vi "TCP_CommModule.vi"(8 "error in (no error)":errorcluster) -> (0 "error out":errorcluster)   [LabVIEW 2021]
uses:
  TCPModuleState.ctl
  TCPCommModuleData.ctl
  TCPQueueData.ctl
  ModelQueueCluster.ctl
  ToModelSourceEnum.ctl
  FromTCPCluster.ctl
  ToModelFromTCPMessage.ctl
  FormControllerToMOdelCluster.ctl
  ToModelFromControllerEnum.ctl
  ToSerialCommand.ctl
  ToSerialCTL.ctl
  QueueEnum.ctl
panel:
  out "bytes written":i32
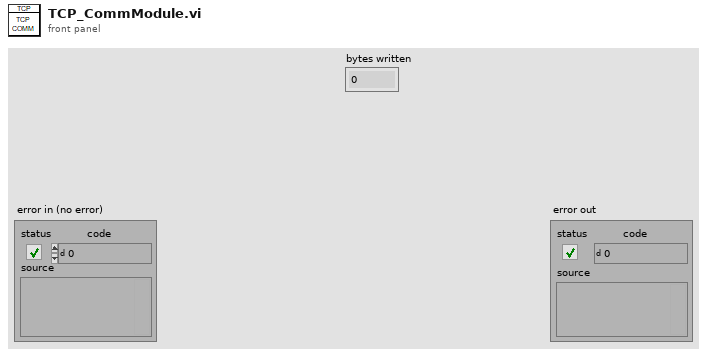
[diagram p1: front panel]
types:
  T1 = typedef "QueueEnum.ctl" = enum16{"Obtain Queue", "Get Queue Ref", "Flush Queue", "Release Queue"}
  T2 = typedef "TCPCommModuleData.ctl" = cluster{"TCP Connection ID":refnum<k5>, "ToTCPModuleQueue":refnum<queue>, "ToModelQueue":refnum<queue>, "Timeout count":u32, "Connected OK?":bool, "ToSerialQueue":refnum<queue>, "VISA resource name":refnum<visa-resource-name>}
  T3 = typedef "TCPModuleState.ctl" = enum16{"Init", "Connect", "Read", "Write", "Disconnect", "ErrorHandler", "Exit"}
  T4 = enum32{"Invalid", "Standard", "Closed", "Hidden", "Minimized", "Maximized"}
  T5 = typedef "TCPQueueData.ctl" = cluster{"Command":T3, "address":string, "remote port":u16, "Data":string}
  T6 = typedef "ModelQueueCluster.ctl" = cluster{"Source":T7, "FromCommunication":T8, "FromControllerCluster":T10}
  T7 = typedef "ToModelSourceEnum.ctl" = enum16{"COM", "TCP", "Controller"}
  T8 = typedef "FromTCPCluster.ctl" = cluster{"Message":T9, "Data":string, "StatusOK?":bool}
  T9 = typedef "ToModelFromTCPMessage.ctl" = enum16{"Exit", "DataWritten", "DataReceived", "Timeout", "UnableToConnect", "Disconnected", "Connected"}
  T10 = typedef "FormControllerToMOdelCluster.ctl" = cluster{"Command":T11, "IP Address":string, "Remote Port":u16, "Data":string, "TCP/COM":bool, "VISA resource name":refnum<visa-resource-name>}
  T11 = typedef "ToModelFromControllerEnum.ctl" = enum16{"StopLogging", "StartLogging", "SlideChange", "SendMessage", "Exit", "Disconnect", "Connect"}
  T12 = enum16{"Standard", "Buffered", "CRLF", "Immediate"}
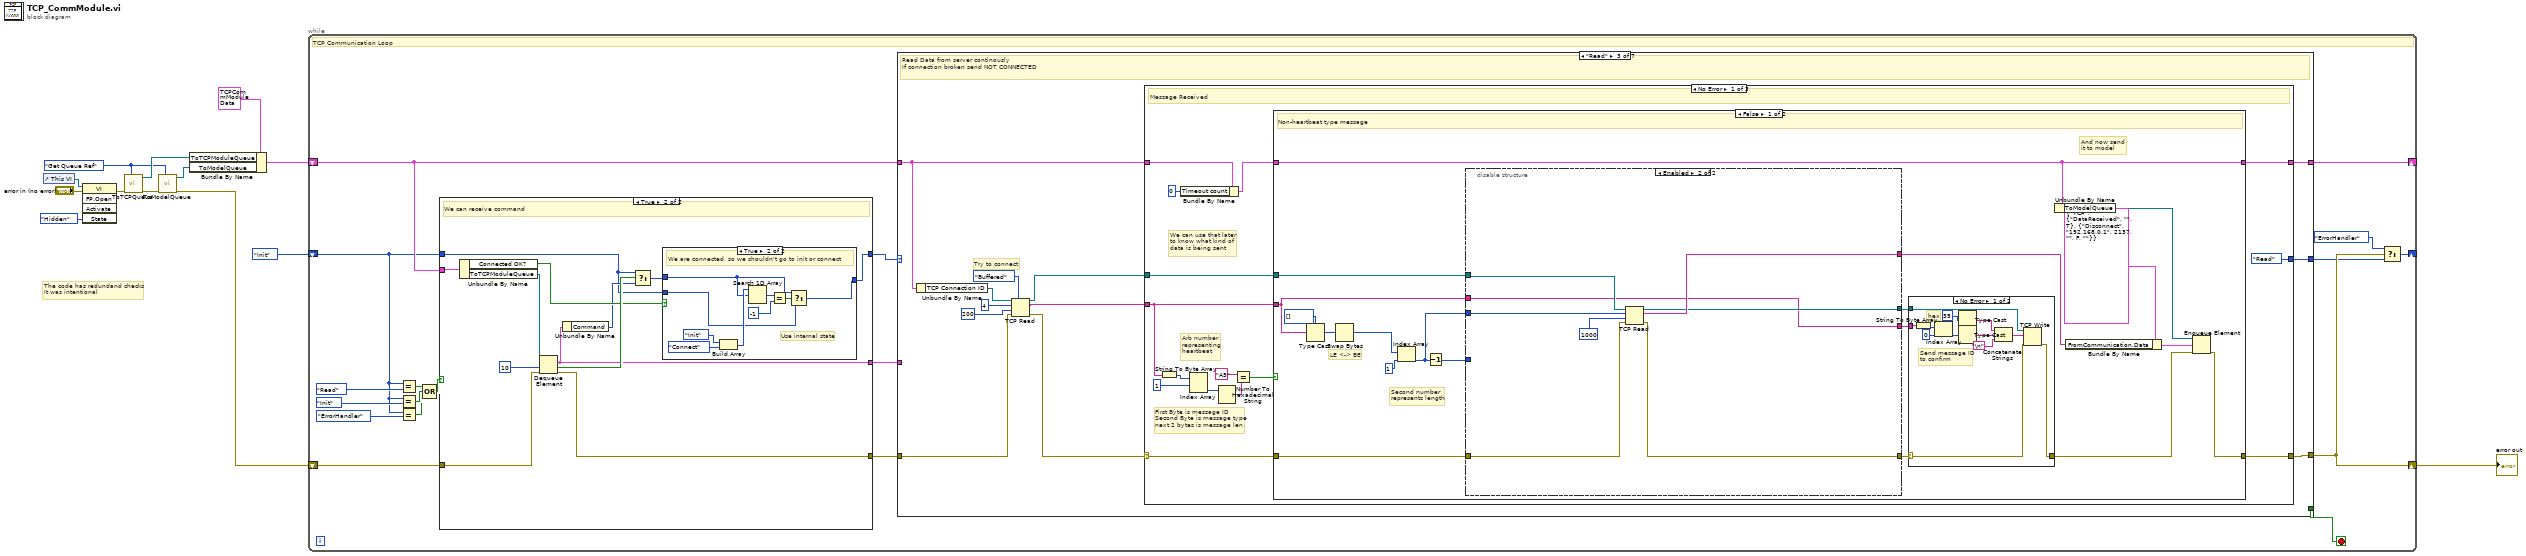
[diagram p0: block diagram]
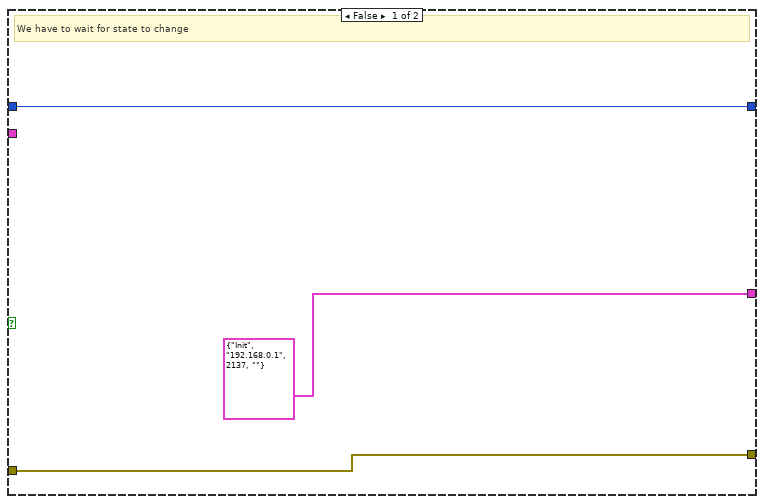
[diagram p2: hidden frame]
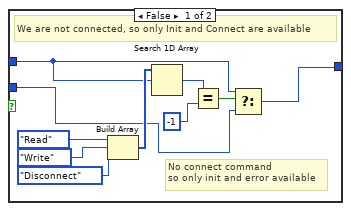
[diagram p3: hidden frame]
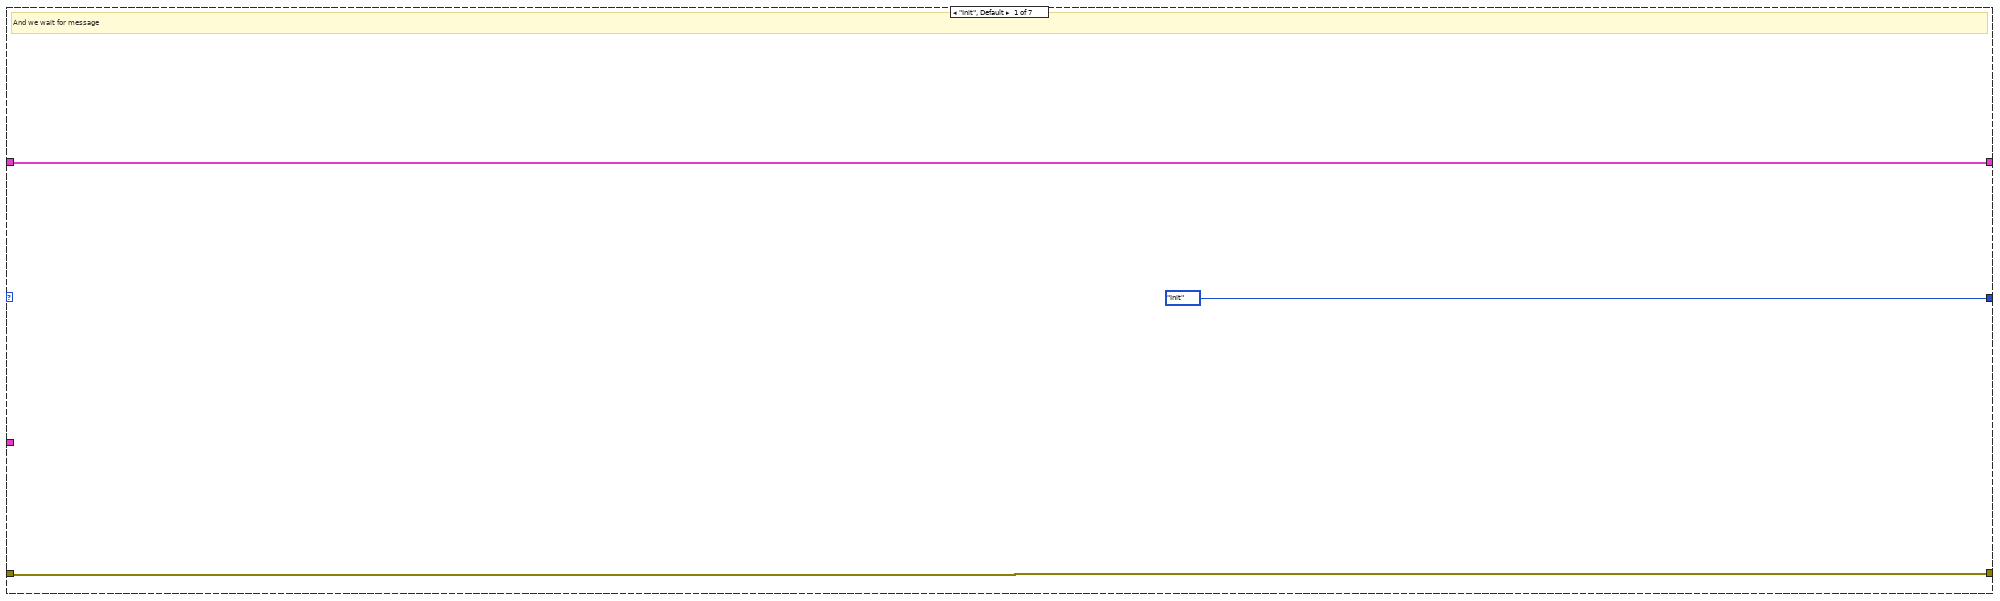
[diagram p4: hidden frame]
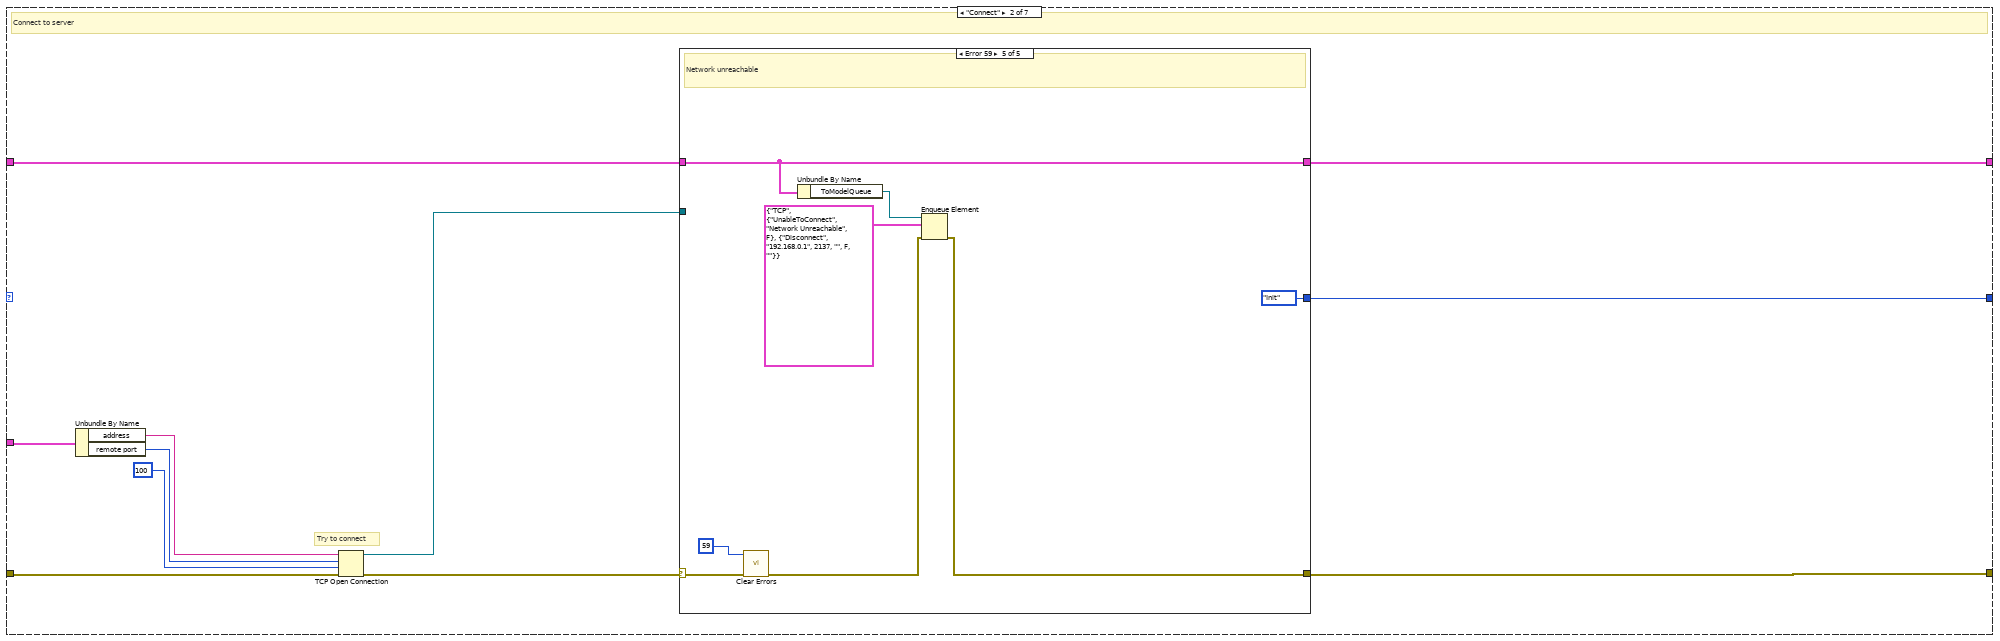
[diagram p5: hidden frame]
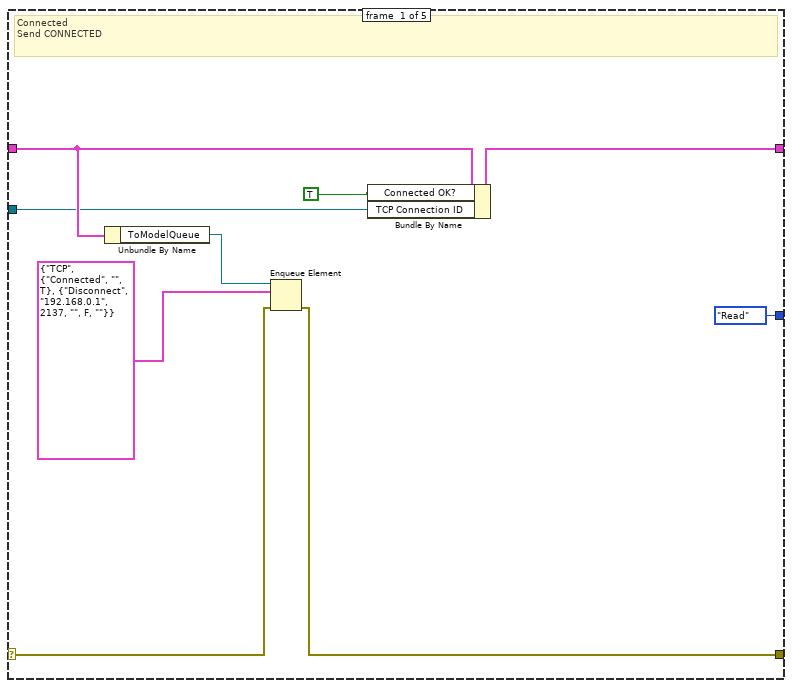
[diagram p6: hidden frame]
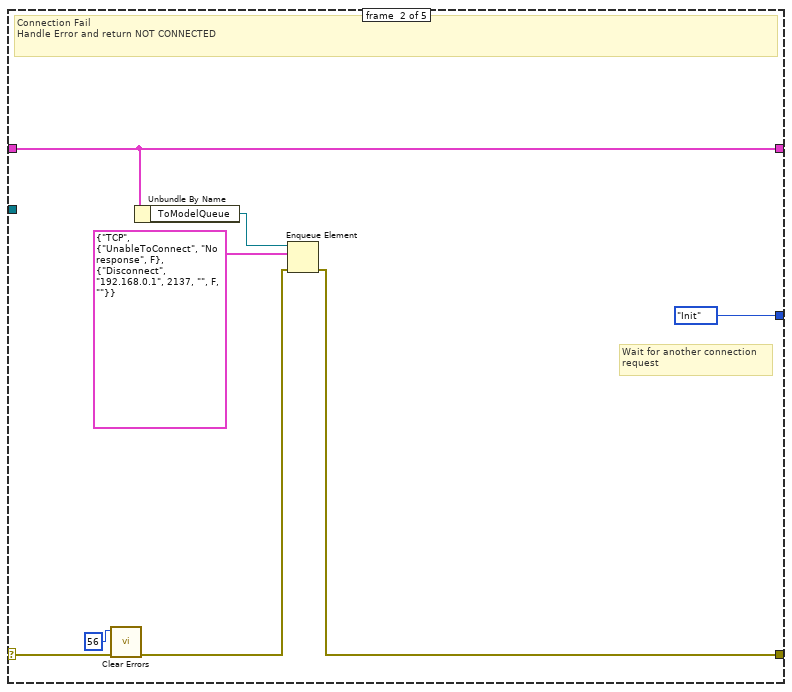
[diagram p7: hidden frame]
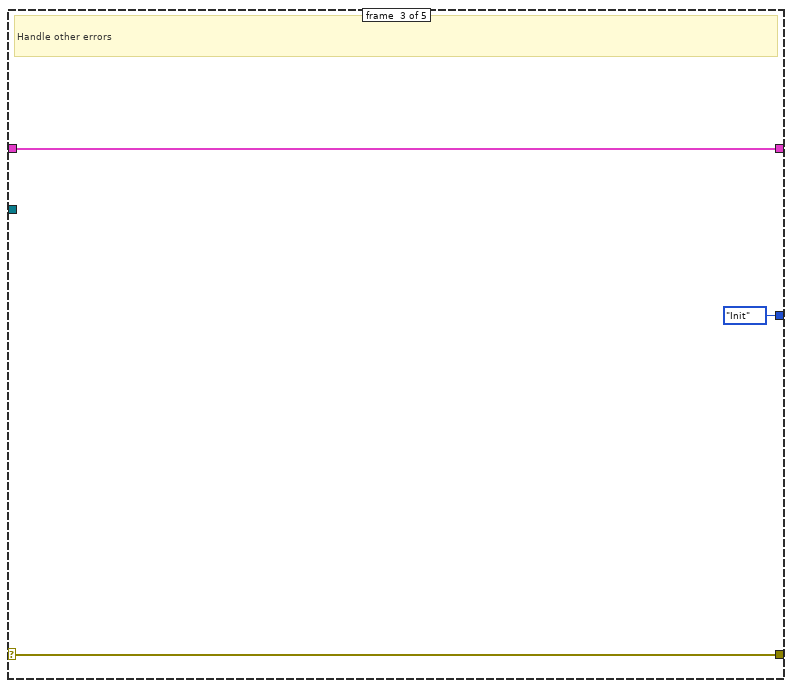
[diagram p8: hidden frame]
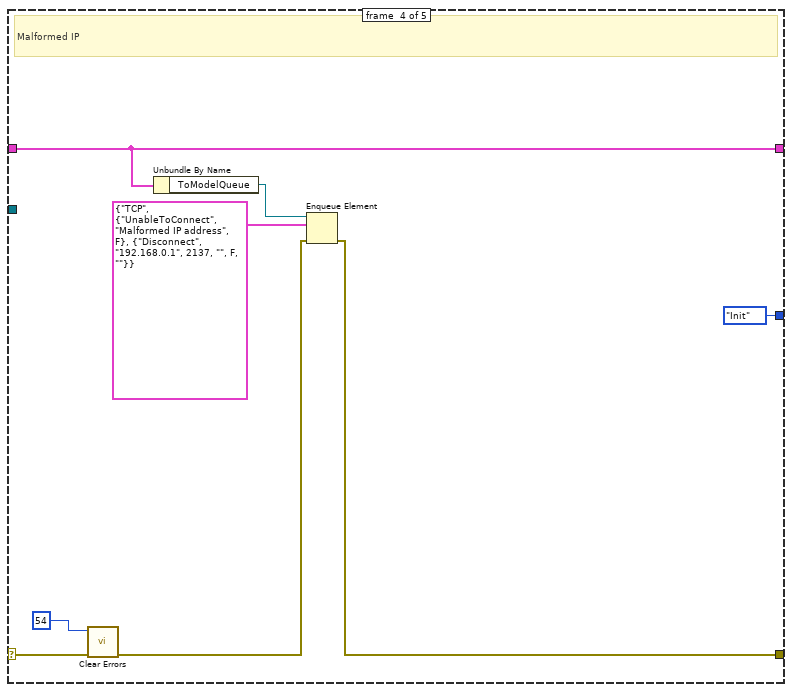
[diagram p9: hidden frame]
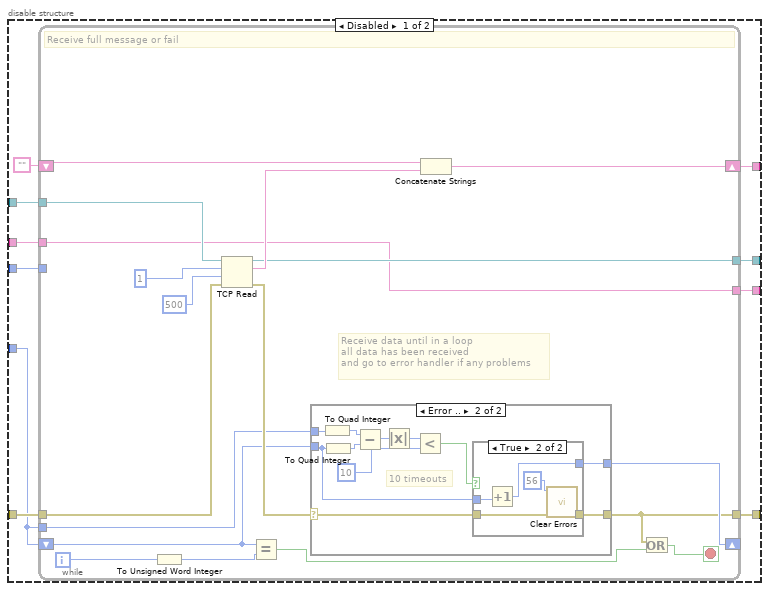
[diagram p11: hidden frame]
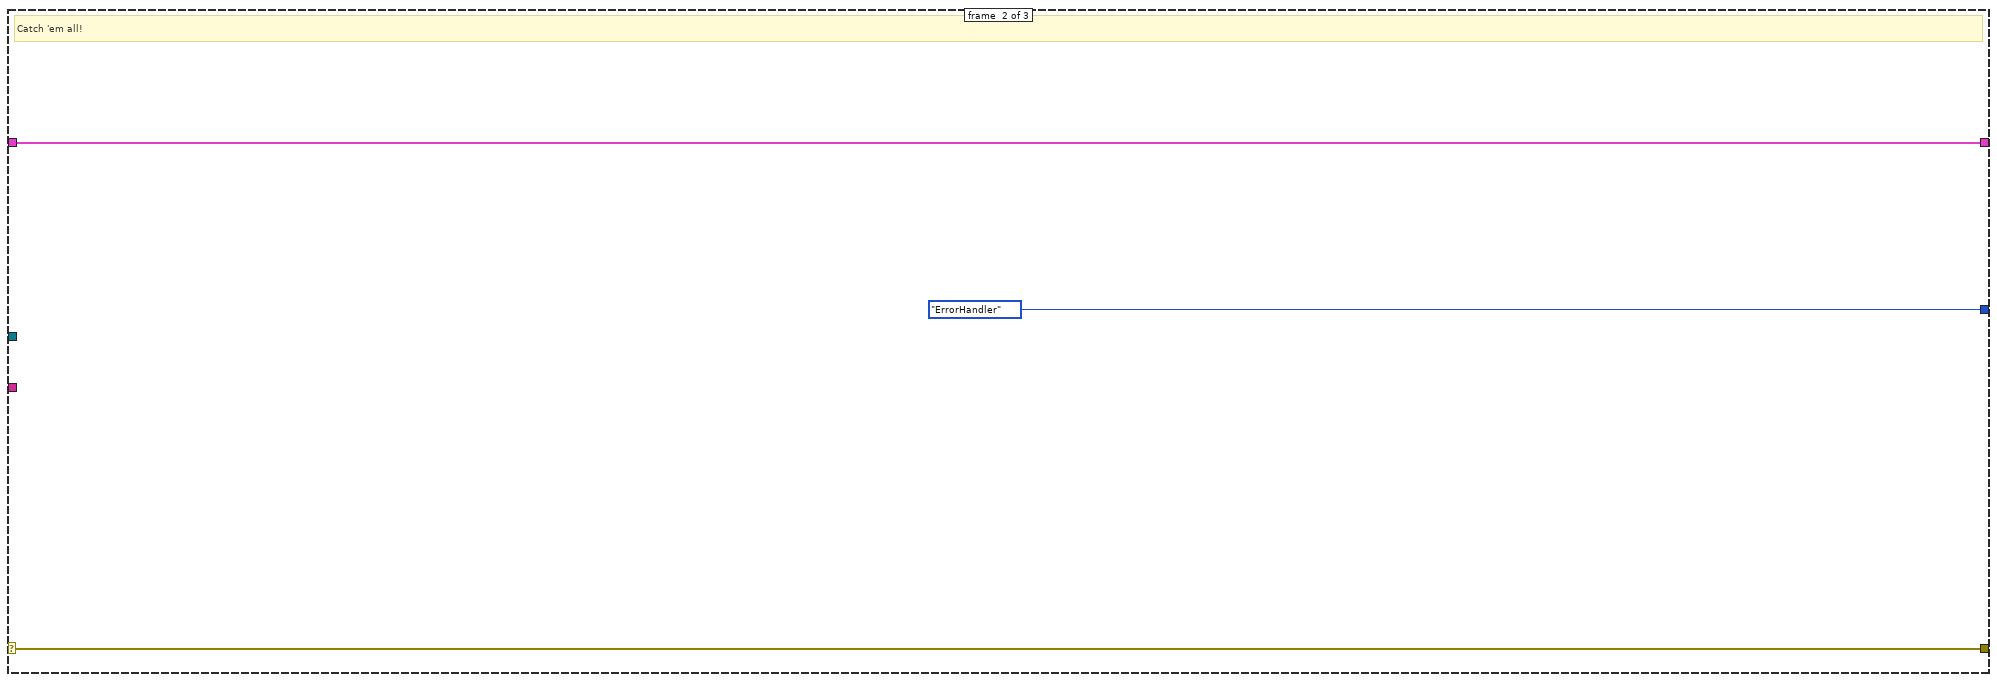
[diagram p15: hidden frame]
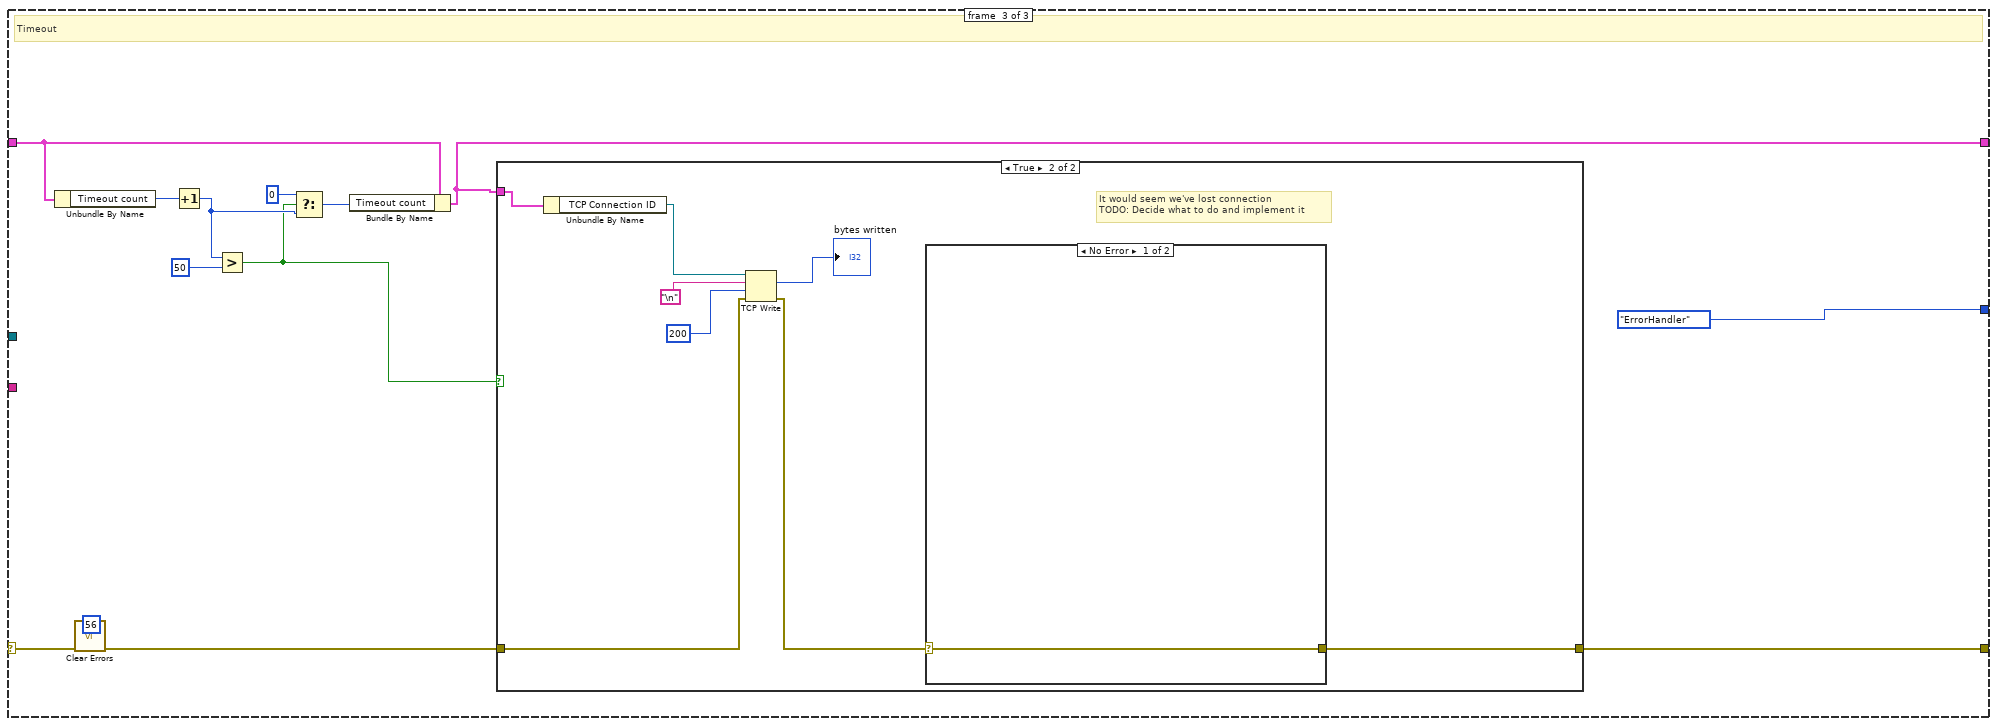
[diagram p16: hidden frame]
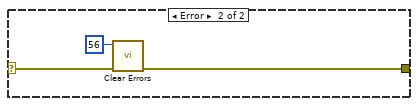
[diagram p18: hidden frame]
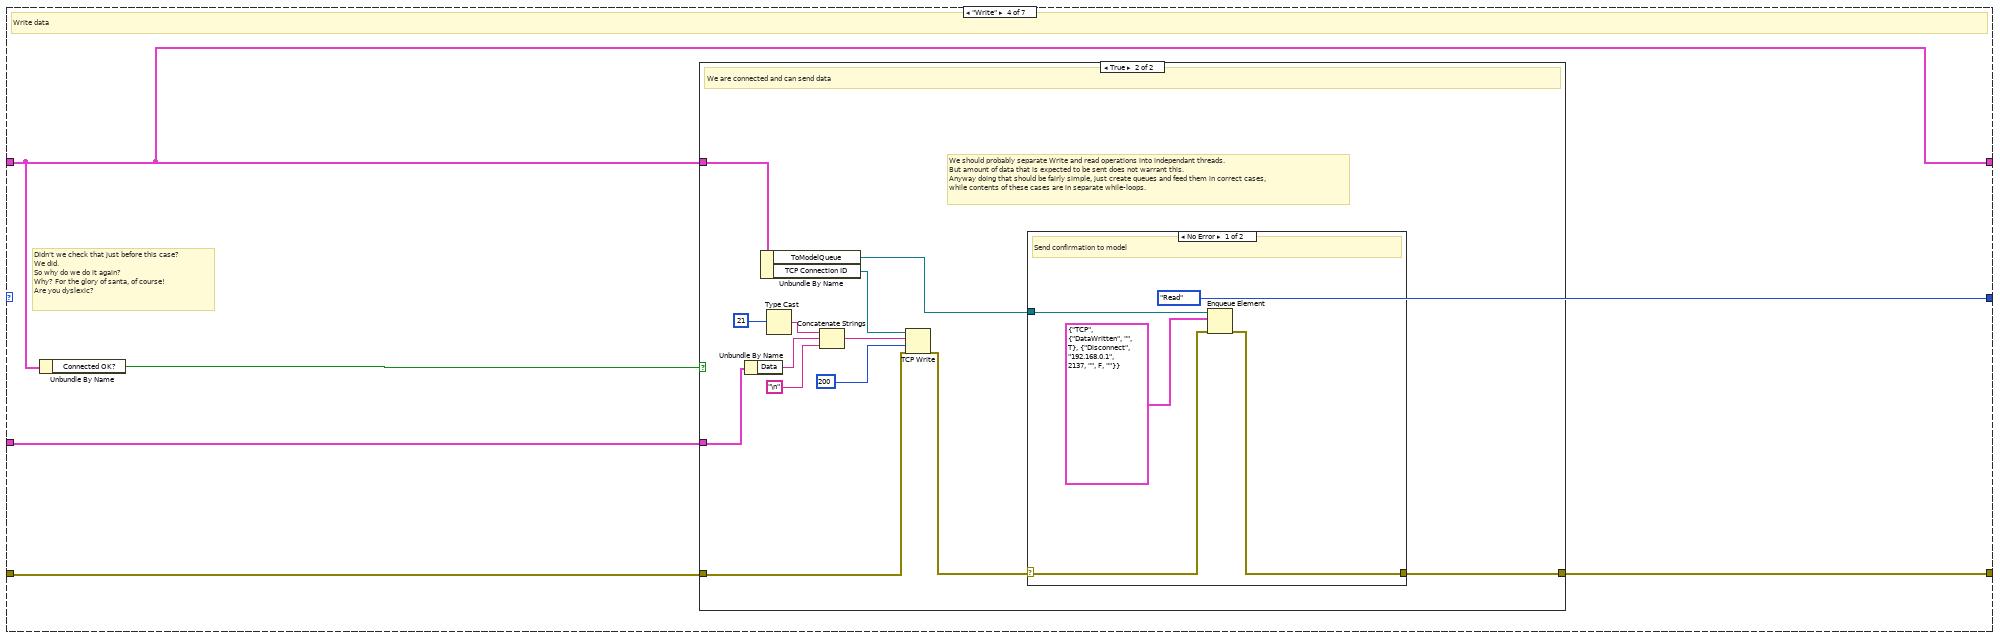
[diagram p19: hidden frame]
diagram:
  w2 = QueueEnum."Get Queue Ref"
  # "The code has redundand checks\nIt was intentional"
  n1 = control-ref of="This VI"() -> (w13:refnum<vi>)
  n2 = invoke class="VI" method="FP.Open"(reference=w13, error in="error in (no error)", "State"=T4."Hidden") -> (error out=w7:errorcluster)  [unwired: 2 in, 4 out]
  n3 = call "ToTCPQueue.vi"("Enum"=w2, "error in (no error)"=w7) -> ("error out"=w6:errorcluster, "queue out"=w5:refnum<queue>)  [unwired: 8 in]
  n4 = call "ToModelQueue.vi"("Enum"=w2, "error in (no error)"=w6) -> ("error out"=w4:errorcluster, "queue out"=w3:refnum<queue>)  [unwired: 8 in]
  n5 = Bundle By Name(cluster=T2 {"TCP Connection ID"=refnum, "ToTCPModuleQueue"=refnum, "ToModelQueue"=refnum, "Timeout count"=0, "Connected OK?"=FALSE, "ToSerialQueue"=refnum, "VISA resource name"=""}, "ToTCPModuleQueue"=w5, "ToModelQueue"=w3) -> (w9:T2)
  n6 = while {
    shift-right: [w25] -> _
    shift-left: TCPModuleState."Init" -> [w14]
    shift-right: [w22] -> _
    shift-left: w9 -> [w27]
    shift-right: [w26] -> w8
    shift-left: w4 -> [w31]
    stop <- w32 stop-if-true
    # "TCP Communication Loop"
    n7 = Equal?(x=w14, y=TCPModuleState."Read") -> (x = y?=w20:bool)
    n8 = Equal?(x=w14, y=TCPModuleState."Init") -> (x = y?=w19:bool)
    n9 = Equal?(x=w14, y=TCPModuleState."ErrorHandler") -> (x = y?=w15:bool)
    n10 = Compound Arithmetic op=OR(w20, w19, w15) -> (w17:bool)
    n11 = case shown="True" w17 {
      tunnel: w31 -> [w35 w47]
      tunnel: [w33 w37] -> w30
      tunnel: [w35 w44] -> w29
      tunnel: [T5 {"Command"=enum."Init", "address"="192.168.0.1", "remote port"=2137, "Data"=""} w42] -> w28
      tunnel: w27 -> [_ w41]
      tunnel: w14 -> [w33 w36]
      frame False {
        # "We have to wait for state to change"
      }
      frame True {
        # "We can receive command"
        n12 = Unbundle By Name(w41) -> ("Connected OK?"=w40:bool, "ToTCPModuleQueue"=w46:refnum<queue>)
        n13 = Dequeue Element(queue=w46, timeout in ms (-1)=10, error in (no error)=w47) -> (element=w42:T5, timed out?=w45:bool, error out=w44:errorcluster)  [unwired: 1 out]
        n14 = Unbundle By Name(w42) -> ("Command"=w39:T3)
        n15 = Select(t=w36, s=w45, f=w39) -> (s? t:f=w38:T3)
        n16 = case shown="True" w40 {
          tunnel: w38 -> [w50 w60]
          tunnel: [w49 w58] -> w37
          tunnel: w36 -> [w48 w59]
          frame False {
            # "No connect command \nso only init and error available"
            # "We are not connected, so only Init and Connect are available"
            n17 = Build Array(TCPModuleState."Read", TCPModuleState."Write", TCPModuleState."Disconnect") -> (w54:T3[])
            n18 = Search 1D Array(1D array=w54, element=w50) -> (index of element=w53:i32)  [unwired: 1 in]
            n19 = Equal?(x=w53, y=-1) -> (x = y?=w51:bool)
            n20 = Select(t=w50, s=w51, f=w48) -> (s? t:f=w49:T3)
          }
          frame True {
            # "Use internal state"
            # "We are connected, so we shouldn't go to init or connect"
            n21 = Build Array(TCPModuleState."Init", TCPModuleState."Connect" ("element")) -> (w64:T3[])
            n22 = Search 1D Array(1D array=w64, element=w60) -> (index of element=w63:i32)  [unwired: 1 in]
            n23 = Equal?(x=w63, y=-1) -> (x = y?=w61:bool)
            n24 = Select(t=w60, s=w61, f=w59) -> (s? t:f=w58:T3)
          }
        }
      }
    }
    n25 = case shown="\"Read\"" w30 {
      tunnel: [_ _ _ _ _ _ TRUE] -> w32
      tunnel: w29 -> [w69 w80 w126 w267 w300 w310 w343]
      tunnel: w28 -> [_ w79 _ w265 _ _ _]
      tunnel: w27 -> [w67 w74 w120 w264 w293 w305 w345]
      tunnel: [w69 w73 w122 w263 w294 w309 w342] -> w26
      tunnel: [TCPModuleState."Init" ("f") w71 w121 TCPModuleState."Read" ("f") TCPModuleState."Init" ("f") w307 TCPModuleState."Exit" ("f")] -> w23
      tunnel: [w67 w72 w119 w264 w292 w304 w345] -> w22
      frame "Init", Default {
        # "And we wait for message"
      }
      frame "Connect" {
        # "Try to connect"
        # "Connect to server"
        n26 = Unbundle By Name(w79) -> ("address"=w78:string, "remote port"=w77:u16)
        n27 = TCP Open Connection(address=w78, remote port or service name=w77, timeout ms (60000)=100, error in (no error)=w80) -> (connection ID=w70:refnum<k5>, error out=w75:errorcluster)  [unwired: 1 in]
        n28 = case shown="Error 59" w75 {
          selector: w75 -> [w87 w96 w99 w107 w115]
          tunnel: w74 -> [w85 w95 w100 w101 w109]
          tunnel: [w86 w91 w99 w102 w110] -> w73
          tunnel: [w83 w95 w100 w101 w109] -> w72
          tunnel: [TCPModuleState."Read" ("f") TCPModuleState."Init" ("f") TCPModuleState."Init" ("f") TCPModuleState."Init" ("f") TCPModuleState."Init" ("f")] -> w71
          tunnel: w70 -> [w81 _ _ _ _]
          frame #0 {
            # "Connected\nSend CONNECTED"
            n29 = Unbundle By Name(w85) -> ("ToModelQueue"=w89:refnum<queue>)
            n30 = Enqueue Element(queue=w89, element=T6 {"Source"=enum."TCP", "FromCommunication"={"Message"=enum."Connected", "Data"="", "StatusOK?"=TRUE}, "FromControllerCluster"={"Command"=enum."Disconnect", "IP Address"="192.168.0.1", "Remote Port"=2137, "Data"="", "TCP/COM"=FALSE, "VISA resource name"=""}}, error in (no error)=w87) -> (error out=w86:errorcluster)  [unwired: 1 in, 2 out]
            n31 = Bundle By Name(cluster=w85, "Connected OK?"=TRUE, "TCP Connection ID"=w81) -> (w83:T2)
          }
          frame #1 {
            # "Wait for another connection\nrequest"
            # "Connection Fail\nHandle Error and return NOT CONNECTED"
            n32 = call <vilib>:"Clear Errors.vi"("error in (no error)"=w96, "specific error code to clear (0: all)"=56) -> ("error out"=w92:errorcluster)  [unwired: 4 in, 1 out]
            n33 = Unbundle By Name(w95) -> ("ToModelQueue"=w94:refnum<queue>)
            n34 = Enqueue Element(queue=w94, element=T6 {"Source"=enum."TCP", "FromCommunication"={"Message"=enum."UnableToConnect", "Data"="No response", "StatusOK?"=FALSE}, "FromControllerCluster"={"Command"=enum."Disconnect", "IP Address"="192.168.0.1", "Remote Port"=2137, "Data"="", "TCP/COM"=FALSE, "VISA resource name"=""}}, error in (no error)=w92) -> (error out=w91:errorcluster)  [unwired: 1 in, 2 out]
          }
          frame #2 {
            # "Handle other errors"
          }
          frame #3 {
            # "Malformed IP"
            n35 = call <vilib>:"Clear Errors.vi"("error in (no error)"=w107, "specific error code to clear (0: all)"=54) -> ("error out"=w103:errorcluster)  [unwired: 4 in, 1 out]
            n36 = Unbundle By Name(w101) -> ("ToModelQueue"=w105:refnum<queue>)
            n37 = Enqueue Element(queue=w105, element=T6 {"Source"=enum."TCP", "FromCommunication"={"Message"=enum."UnableToConnect", "Data"="Malformed IP address", "StatusOK?"=FALSE}, "FromControllerCluster"={"Command"=enum."Disconnect", "IP Address"="192.168.0.1", "Remote Port"=2137, "Data"="", "TCP/COM"=FALSE, "VISA resource name"=""}}, error in (no error)=w103) -> (error out=w102:errorcluster)  [unwired: 1 in, 2 out]
          }
          frame #4 {
            # "Network unreachable"
            n38 = call <vilib>:"Clear Errors.vi"("error in (no error)"=w115, "specific error code to clear (0: all)"=59) -> ("error out"=w111:errorcluster)  [unwired: 4 in, 1 out]
            n39 = Unbundle By Name(w109) -> ("ToModelQueue"=w113:refnum<queue>)
            n40 = Enqueue Element(queue=w113, element=T6 {"Source"=enum."TCP", "FromCommunication"={"Message"=enum."UnableToConnect", "Data"="Network Unreachable", "StatusOK?"=FALSE}, "FromControllerCluster"={"Command"=enum."Disconnect", "IP Address"="192.168.0.1", "Remote Port"=2137, "Data"="", "TCP/COM"=FALSE, "VISA resource name"=""}}, error in (no error)=w111) -> (error out=w110:errorcluster)  [unwired: 1 in, 2 out]
          }
        }
      }
      frame "Read" {
        # "Try to connect"
        # "Read Data from server continously\nIf connection broken send NOT CONNECTED"
        n41 = Unbundle By Name(w120) -> ("TCP Connection ID"=w128:refnum<k5>)
        n42 = TCP Read(connection ID=w128, bytes to read=4, error in (no error)=w126, 7:T12."Buffered" ("mode (standard)"), 9:200 ("timeout ms (25000)")) -> (connection ID out=w123:refnum<k5>, data out=w117:string, error out=w124:errorcluster)
        n43 = case shown="No Error" w124 {
          selector: w124 -> [w133 w236 w248]
          tunnel: w123 -> [w134 _ _]
          tunnel: [w140 w236 w241] -> w122
          tunnel: [TCPModuleState."Read" TCPModuleState."ErrorHandler" TCPModuleState."ErrorHandler"] -> w121
          tunnel: w120 -> [w137 w234 w245]
          tunnel: [w138 w234 w243] -> w119
          tunnel: w117 -> [w129 _ _]
          frame #0 {
            # "First Byte is message ID\nSecond Byte is message type\nnext 2 bytes is message len"
            # "We can use that later \nto know what kind of\ndata is being sent"
            # "Arb number\nrepresenting\nheartbeat"
            # "Message Received"
            n44 = String To Byte Array(string=w129) -> (unsigned byte array=w132:u8[])
            n45 = Bundle By Name(cluster=w137, "Timeout count"=u32 0) -> (w136:T2)
            n46 = Index Array(array=w132, index #1=1 ("index")) -> (element #2=w130:u8)  [unwired: 1 in, 1 out]
            n47 = Number To Hexadecimal String(2:w130) -> (0:w143:string)  [unwired: 1 in]
            n48 = Equal?(x="A5", y=w143) -> (x = y?=w141:bool)
            n49 = case shown="False" w141 {
              tunnel: w133 -> [w154 w233]
              tunnel: [w159 w233] -> w140
              tunnel: w134 -> [w155 _]
              tunnel: w136 -> [w161 w232]
              tunnel: [w161 w232] -> w138
              tunnel: w129 -> [w149 _]
              frame False {
                # "LE <-> BE"
                # "Second number\nrepresents length"
                # "And now send\nit to model"
                # "Non-heartbeat type message"
                n50 = Type Cast(type=u16[] [], x=w149) -> (*(type *) &x=w151:u16[])
                n51 = Swap Bytes(anything=w151) -> (byte swapped=w150:u16[])
                n52 = Index Array(array=w150, index=1) -> (element=w148:u16)
                n53 = Decrement(x=w148) -> (x-1=w153:u16)
                n54 = disable-structure shown="Enabled" {
                  disable-tunnel: w153 -> [w181 _]
                  disable-tunnel: [w176 w226] -> w147
                  disable-tunnel: [w185 w228] -> w157
                  disable-tunnel: w154 -> [w184 w229]
                  disable-tunnel: w155 -> [w183 w230]
                  disable-tunnel: w149 -> [w180 w224]
                  disable-tunnel: w148 -> [w179 w227]
                  disable-tunnel: [w178 w224] -> w145
                  disable-tunnel: [w177 w225] -> w144
                  frame Disabled {
                    n55 = while {
                      tunnel: w184 -> [w203]
                      tunnel: [w190] -> w176
                      tunnel: w183 -> [w202]
                      shift-right: [w198] -> w185
                      shift-left: "" -> [w200]
                      tunnel: [w197] -> w177
                      shift-right: [w191] -> _
                      shift-left: w181 -> [w192]
                      tunnel: w181 -> [w193]
                      tunnel: [w187] -> w178
                      tunnel: w180 -> [w187]
                      tunnel: w179 -> [_]
                      i -> [w196]
                      stop <- w189 stop-if-true
                      # "Receive data until in a loop\nall data has been received\nand go to error handler if any problems"
                      # "Receive full message or fail"
                      n56 = To Unsigned Word Integer(number=w196) -> (unsigned 16bit integer=w195:u16)
                      n57 = TCP Read(connection ID=w202, bytes to read=1, error in (no error)=w203, 9:500 ("timeout ms (25000)")) -> (connection ID out=w197:refnum<k5>, data out=w199:string, error out=w194:errorcluster)  [unwired: 1 in]
                      n58 = Equal?(x=w192, y=w195) -> (x = y?=w188:bool)
                      n59 = case shown="Error .." w194 {
                        selector: w194 -> [w205 w216]
                        tunnel: [w205 w215] -> w190
                        tunnel: w193 -> [_ w213]
                        tunnel: w192 -> [w204 w207]
                        tunnel: [w204 w206] -> w191
                        frame No Error {
                        }
                        frame Error {
                          # "10 timeouts"
                          n60 = To Quad Integer(1:w213) -> (0:w212:i64)
                          n61 = To Quad Integer(1:w207) -> (0:w211:i64)
                          n62 = Subtract(x=w212, y=w211) -> (x-y=w214:i64)
                          n63 = Absolute Value(x=w214) -> (abs(x)=w210:i64)
                          n64 = Less?(x=w210, y=i64 10) -> (x < y?=w208:bool)
                          n65 = case shown="True" w208 {
                            tunnel: w216 -> [w218 w222]
                            tunnel: [w218 w221] -> w215
                            tunnel: w207 -> [w217 w220]
                            tunnel: [w217 w219] -> w206
                            frame False {
                            }
                            frame True {
                              n66 = Increment(x=w220) -> (x+1=w219:u16)
                              n67 = call <vilib>:"Clear Errors.vi"("error in (no error)"=w222, "specific error code to clear (0: all)"=56) -> ("error out"=w221:errorcluster)  [unwired: 4 in, 1 out]
                            }
                          }
                        }
                      }
                      n68 = Concatenate Strings(w200, w199) -> (w198:string)
                      n69 = Or(x=w190, y=w188) -> (x .or. y?=w189:bool)
                    }
                  }
                  frame Enabled {
                    n70 = TCP Read(connection ID=w230, bytes to read=w227, error in (no error)=w229, 9:1000 ("timeout ms (25000)")) -> (connection ID out=w225:refnum<k5>, data out=w228:string, error out=w226:errorcluster)  [unwired: 1 in]
                  }
                }
                n71 = case shown="No Error" w147 {
                  selector: w147 -> [w169 w175]
                  tunnel: w145 -> [w174 _]
                  tunnel: w144 -> [w170 _]
                  tunnel: [w168 w175] -> w146
                  frame No Error {
                    # "hex"
                    # "Send message ID\nto confirm"
                    n72 = String To Byte Array(string=w174) -> (unsigned byte array=w173:u8[])
                    n73 = Index Array(array=w173, index=0) -> (element=w171:u8)
                    n74 = Type Cast(x=w171) -> (*(type *) &x=w167:string)  [unwired: 1 in]
                    n75 = Type Cast(x=u8 35) -> (*(type *) &x=w163:string)  [unwired: 1 in]
                    n76 = Concatenate Strings(w163, w167, "\n") -> (w166:string)
                    n77 = TCP Write(connection ID=w170, data in=w166, error in (no error)=w169) -> (error out=w168:errorcluster)  [unwired: 1 in, 2 out]
                  }
                  frame Error {
                    # "Decide how to handle\nmessage not received"
                  }
                }
                n78 = Unbundle By Name(w161) -> ("ToModelQueue"=w160:refnum<queue>)
                n79 = Bundle By Name(cluster=T6 {"Source"=enum."TCP", "FromCommunication"={"Message"=enum."DataReceived", "Data"="", "StatusOK?"=TRUE}, "FromControllerCluster"={"Command"=enum."Disconnect", "IP Address"="192.168.0.1", "Remote Port"=2137, "Data"="", "TCP/COM"=FALSE, "VISA resource name"=""}} ("element"), "FromCommunication.Data"=w157) -> (w156:T6)
                n80 = Enqueue Element(queue=w160, element=w156, error in (no error)=w146) -> (error out=w159:errorcluster)  [unwired: 1 in, 2 out]
              }
              frame True {
                # "We can check here if device is alive\nDevice should send periodic heartbeat messages.\nThough in this particular project we expect\ncontinous data flow from ToF sensors so this is redundant.\nBut can be useful in future."
                # "Heartbeat\nContinue"
              }
            }
          }
          frame #1 {
            # "Catch 'em all!"
          }
          frame #2 {
            # "Timeout"
            n81 = Unbundle By Name(w245) -> ("Timeout count"=w246:u32)
            n82 = call <vilib>:"Clear Errors.vi"("error in (no error)"=w248, "specific error code to clear (0: all)"=56) -> ("error out"=w242:errorcluster)  [unwired: 4 in, 1 out]
            n83 = Increment(x=w246) -> (x+1=w239:u32)
            n84 = Greater?(x=w239, y=u32 50) -> (0:w237:bool)
            n85 = Select(t=u32 0, s=w237, f=w239) -> (s? t:f=w240:u32)
            n86 = Bundle By Name(cluster=w245, "Timeout count"=w240) -> (w243:T2)
            n87 = case shown="True" w237 {
              tunnel: w243 -> [_ w258]
              tunnel: w242 -> [w250 w256]
              tunnel: [w250 w253] -> w241
              frame False {
              }
              frame True {
                # "It would seem we've lost connection\nTODO: Decide what to do and implement it"
                n88 = Unbundle By Name(w258) -> ("TCP Connection ID"=w257:refnum<k5>)
                n89 = TCP Write(connection ID=w257, data in="\n", error in (no error)=w256, 9:200 ("timeout ms (25000)")) -> (bytes written=→"bytes written":i32, error out=w254:errorcluster)  [unwired: 1 out]
                n90 = case shown="No Error" w254 {
                  selector: w254 -> [w259 w262]
                  tunnel: [w259 w261] -> w253
                  frame No Error {
                  }
                  frame Error {
                    n91 = call <vilib>:"Clear Errors.vi"("error in (no error)"=w262, "specific error code to clear (0: all)"=56) -> ("error out"=w261:errorcluster)  [unwired: 4 in, 1 out]
                  }
                }
              }
            }
          }
        }
      }
      frame "Write" {
        # "Didn't we check that just before this case?\nWe did.\nSo why do we do it again?\nWhy? For the glory of santa, of course!\nAre you dyslexic?"
        # "Write data"
        n92 = Unbundle By Name(w264) -> ("Connected OK?"=w266:bool)
        n93 = case shown="True" w266 {
          tunnel: w267 -> [w269 w280]
          tunnel: w264 -> [_ w282]
          tunnel: w265 -> [_ w278]
          tunnel: [w269 w276] -> w263
          frame False {
            # "Why are we here? Ignore!"
          }
          frame True {
            # "We should probably separate Write and read operations into independant threads.\nBut amount of data that is expected to be sent does not warrant this.\nAnyway doing that should be fairly simple, just create queues and feed them in correct cases,\nwhile contents of these cases are in separate while-loops."
            # "We are connected and can send data"
            n94 = Unbundle By Name(w278) -> ("Data"=w274:string)
            n95 = Unbundle By Name(w282) -> ("ToModelQueue"=w275:refnum<queue>, "TCP Connection ID"=w281:refnum<k5>)
            n96 = Type Cast(x=u8 21) -> (*(type *) &x=w270:string)  [unwired: 1 in]
            n97 = Concatenate Strings(w270, w274, "\n") -> (w273:string)
            n98 = TCP Write(connection ID=w281, data in=w273, error in (no error)=w280, 9:200 ("timeout ms (25000)")) -> (error out=w277:errorcluster)  [unwired: 2 out]
            n99 = case shown="No Error" w277 {
              selector: w277 -> [w285 w289]
              tunnel: [w284 w288] -> w276
              tunnel: w275 -> [w286 w290]
              frame No Error {
                # "Send confirmation to model"
                n100 = Enqueue Element(queue=w286, element=T6 {"Source"=enum."TCP", "FromCommunication"={"Message"=enum."DataWritten", "Data"="", "StatusOK?"=TRUE}, "FromControllerCluster"={"Command"=enum."Disconnect", "IP Address"="192.168.0.1", "Remote Port"=2137, "Data"="", "TCP/COM"=FALSE, "VISA resource name"=""}}, error in (no error)=w285) -> (error out=w284:errorcluster)  [unwired: 1 in, 2 out]
              }
              frame Error, Default {
                # "Send confirmation of failure to model"
                n101 = Enqueue Element(queue=w290, element=T6 {"Source"=enum."TCP", "FromCommunication"={"Message"=enum."DataWritten", "Data"="", "StatusOK?"=FALSE}, "FromControllerCluster"={"Command"=enum."Disconnect", "IP Address"="192.168.0.1", "Remote Port"=2137, "Data"="", "TCP/COM"=FALSE, "VISA resource name"=""}}, error in (no error)=w289) -> (error out=w288:errorcluster)  [unwired: 1 in, 2 out]
              }
            }
          }
        }
      }
      frame "Disconnect" {
        # "Update connection status"
        # "Send message to model"
        # "Try to disconnect"
        # "We were disconnected either way"
        # "After disconnection lets go to init and wait for orders"
        n102 = Unbundle By Name(w293) -> ("ToModelQueue"=w299:refnum<queue>, "TCP Connection ID"=w301:refnum<k5>)
        n103 = TCP Close Connection(connection ID=w301, error in (no error)=w300) -> (error out=w296:errorcluster)  [unwired: 1 in, 1 out]
        n104 = case shown="Error .." w296 {
          tunnel: [TRUE _] -> w297
          frame No Error {
          }
          frame Error {
          }
        }
        n105 = Bundle By Name(cluster=T6 {"Source"=enum."TCP", "FromCommunication"={"Message"=enum."Disconnected", "Data"="", "StatusOK?"=FALSE}, "FromControllerCluster"={"Command"=enum."Disconnect", "IP Address"="192.168.0.1", "Remote Port"=2137, "Data"="", "TCP/COM"=FALSE, "VISA resource name"=""}} ("element"), "FromCommunication.StatusOK?"=w297) -> (w295:T6)
        n106 = Enqueue Element(queue=w299, element=w295, error in (no error)=w296) -> (error out=w294:errorcluster)  [unwired: 1 in, 2 out]
        n107 = Bundle By Name(cluster=w293, "Connected OK?"=FALSE) -> (w292:T2)
      }
      frame "ErrorHandler" {
        # "We should always be able to recover\nIf we did not then we send exit request to model\nLet's wait for a message"
        n108 = case shown="Error 66" w310 {
          selector: w310 -> [w313 w316 w319 w333 w340]
          tunnel: [w313 w316 w320 w325 w337] -> w309
          tunnel: [TCPModuleState."Read" ("f") TCPModuleState."Read" ("f") TCPModuleState."Read" ("f") TCPModuleState."Init" ("f") TCPModuleState."Init" ("f")] -> w306
          tunnel: w305 -> [w311 w314 w317 w324 w336]
          tunnel: [w311 w314 w317 w322 w334] -> w304
          frame #0 {
            # "Handle other errors"
          }
          frame #1 {
          }
          frame #2 {
            # "Handle Timeout"
            n109 = call <vilib>:"Clear Errors.vi"("error in (no error)"=w319, "specific error code to clear (0: all)"=56) -> ("error out"=w320:errorcluster)  [unwired: 4 in, 1 out]
          }
          frame #3 {
            n110 = call <vilib>:"Clear Errors.vi"("error in (no error)"=w333, "specific error code to clear (0: all)"=66) -> ("error out"=w330:errorcluster)  [unwired: 4 in, 1 out]
            n111 = Bundle By Name(cluster=w324, "Connected OK?"=FALSE) -> (w322:T2)
            n112 = call "ToModelQueue.vi"("Enum"=QueueEnum."Get Queue Ref", "error in (no error)"=w330) -> ("error out"=w328:errorcluster, "queue out"=w327:refnum<queue>)  [unwired: 8 in]
            n113 = Enqueue Element(queue=w327, element=T6 {"Source"=enum."TCP", "FromCommunication"={"Message"=enum."Disconnected", "Data"="", "StatusOK?"=FALSE}, "FromControllerCluster"={"Command"=enum."Disconnect", "IP Address"="192.168.0.1", "Remote Port"=2137, "Data"="", "TCP/COM"=FALSE, "VISA resource name"=""}}, error in (no error)=w328) -> (error out=w325:errorcluster)  [unwired: 1 in, 2 out]
          }
          frame #4 {
            # "Tried to connect but nework unreachable"
            n114 = call <vilib>:"Clear Errors.vi"("error in (no error)"=w340, "specific error code to clear (0: all)"=59) -> ("error out"=w337:errorcluster)  [unwired: 4 in, 1 out]
            n115 = Bundle By Name(cluster=w336, "Connected OK?"=FALSE) -> (w334:T2)
          }
        }
        n116 = Select(t=TCPModuleState."ErrorHandler", s=w309, f=w306) -> (s? t:f=w307:T3)
      }
      frame "Exit" {
        # "Exit"
        n117 = Unbundle By Name(w345) -> ("ToModelQueue"=w344:refnum<queue>)
        n118 = Enqueue Element(queue=w344, element=T6 {"Source"=enum."TCP", "FromCommunication"={"Message"=enum."Exit", "Data"="", "StatusOK?"=TRUE}, "FromControllerCluster"={"Command"=enum."Disconnect", "IP Address"="192.168.0.1", "Remote Port"=2137, "Data"="", "TCP/COM"=FALSE, "VISA resource name"=""}}, error in (no error)=w343) -> (error out=w342:errorcluster)  [unwired: 1 in, 2 out]
      }
    }
    n119 = Select(t=TCPModuleState."ErrorHandler", s=w26, f=w23) -> (s? t:f=w25:T3)
  }
  "error out" <- w8
